vi "AxisWriteValues.vi"(1 "AxisNo":u16) -> (0 "AxisWriteValuesOUT":T1={"AxisTarget"=0.0, "AxisTargetVel"=1.0, "AxisStartReq"=FALSE, "AxisStopReq"=FALSE, "AxisClearReq"=FALSE, "AxisMovetype"=FALSE, "AxisMotorON"=FALSE, "MoveModeControl"=0, "AxisHomingVel"=1.0, "AxisAccDecc"=30.0} {"MoveModeControl" items=["Absolute"=1, "Relative"=2, "Velocity"=3, "Homing"=4, "none"=0]})   [LabVIEW 2020, in "SMCD14_lib.lvlib"]
uses:
  AxisWriteValues_typedef.ctl
  Globals.vi
  SMCD14_lib.lvlib
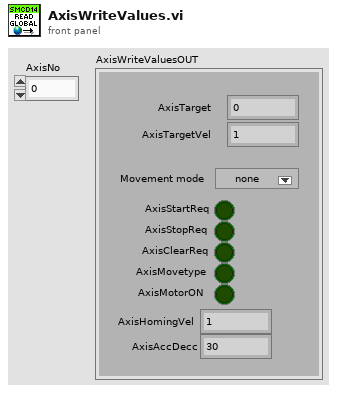
[diagram p1: front panel]
types:
  T1 = typedef "SMCD14_lib.lvlib/AxisWriteValues_typedef.ctl" = cluster{"AxisTarget":dbl, "AxisTargetVel":dbl, "AxisStartReq":bool, "AxisStopReq":bool, "AxisClearReq":bool, "AxisMovetype":bool, "AxisMotorON":bool, "MoveModeControl":u16, "AxisHomingVel":dbl, "AxisAccDecc":dbl}
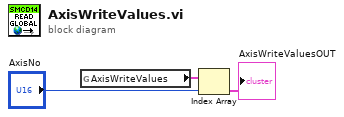
[diagram p0: block diagram]
diagram:
  n1 = global read "Globals.vi" "AxisWriteValues"() -> (w2:T1[])
  n2 = Index Array(array=w2, index="AxisNo") -> (element=→"AxisWriteValuesOUT":T1)
